vi "GetGripLimitSwitches.vi"() -> (2 "Close Limit Switch":bool, 3 "Open Limit Switch":bool)   [LabVIEW 2018]
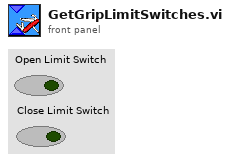
[diagram p1: front panel]
types:
  T1 = typedef "WPI_DigitalInputDevRef.ctl" = cluster{"DevStatus":errorcluster, "DIO Channel":T2}
  T2 = typedef "FPGA_DIOChannel.ctl" = enum8{"DIO 0", "DIO 1", "DIO 2", "DIO 3", "DIO 4", "DIO 5", "DIO 6", "DIO 7", "DIO 8", "DIO 9", "DIO MXP 0", "DIO MXP 1", "DIO MXP 2", "DIO MXP 3", "DIO MXP 4", "DIO MXP 5", "DIO MXP 6", "DIO MXP 7", "DIO MXP 8", "DIO MXP 9", "DIO MXP 10", "DIO MXP 11", "DIO MXP 12", "DIO MXP 13", "DIO MXP 14", "DIO MXP 15", "SPI Port CS1", "SPI Port CS2", "SPI Port CS3", "SPI Port MISO", "SPI Port MOSI", "Invalid"}
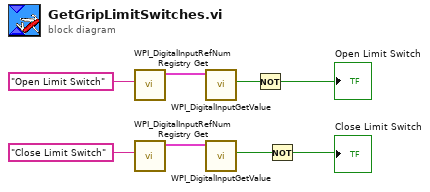
[diagram p0: block diagram]
diagram:
  n1 = call <vilib>:"WPI_DigitalInputRefNum Registry Get.vi"("refnum name"="Open Limit Switch") -> ("DigitalInputDevRef"=w8:T1)  [unwired: 9 in, 1 out]
  n2 = call <vilib>:"WPI_DigitalInputRefNum Registry Get.vi"("refnum name"="Close Limit Switch") -> ("DigitalInputDevRef"=w6:T1)  [unwired: 9 in, 1 out]
  n3 = call <vilib>:"WPI_DigitalInputGetValue.vi"("DigitalInputDevRef"=w8) -> ("Value"=w3:bool)  [unwired: 8 in, 2 out]
  n4 = call <vilib>:"WPI_DigitalInputGetValue.vi"("DigitalInputDevRef"=w6) -> ("Value"=w4:bool)  [unwired: 8 in, 2 out]
  n5 = Not(x=w3) -> (.not. x?=→"Open Limit Switch":bool)
  n6 = Not(x=w4) -> (.not. x?=→"Close Limit Switch":bool)
